vi "fill-lstm-template.vi"() -> ()   [LabVIEW 2020]
uses:
  <vilib>/Analysis/7linalg.llb/Real Transpose Matrix.vi
  <vilib>/Analysis/NI_AALPro.lvlib
panel:
  in  "weight path":path
  in  "name":string
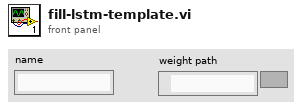
[diagram p1: front panel]
types:
  T1 = typedef "NI_Matrix.lvlib/RealMatrix.ctl" = dbl[][]
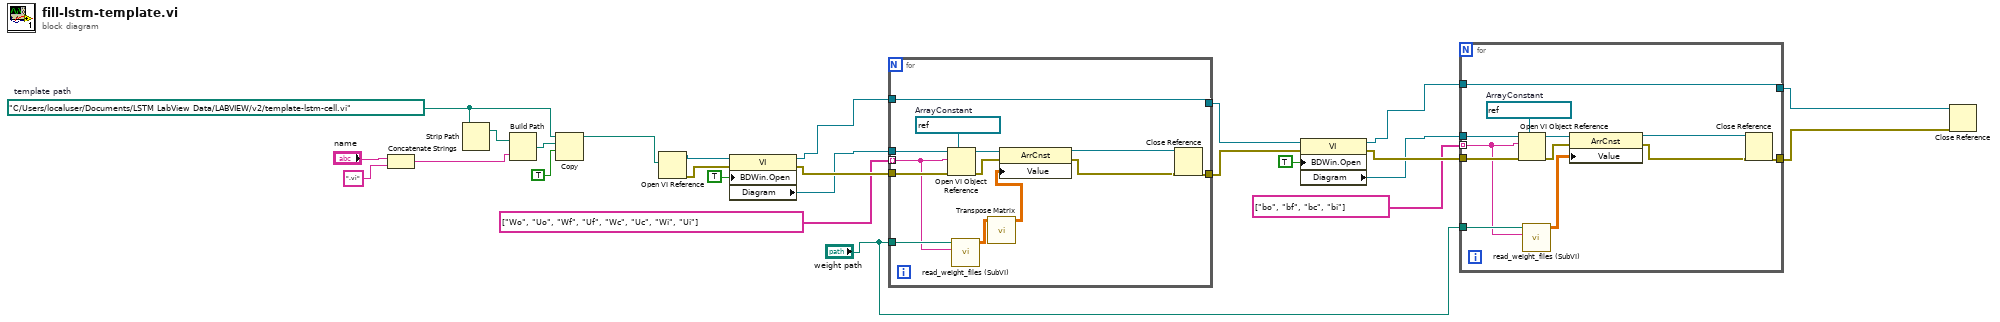
[diagram p0: block diagram]
diagram:
  w18 = path "C:/Users/localuser/Documents/LSTM LabView Data/LABVIEW/v2/template-lstm-cell.vi"  # template path
  n1 = Concatenate Strings("name", ".vi") -> (w20:string)
  n2 = Strip Path(path=w18) -> (stripped path=w23:path)  [unwired: 1 out]
  n3 = Build Path(base path=w23, name or relative path=w20) -> (appended path=w19:path)
  n4 = Copy(9:TRUE, 10:w19, 11:w18) -> (3:w14:path)  [unwired: 2 in, 2 out]
  n5 = Open VI Reference(vi path=w14) -> (vi reference=w16:refnum<vi>, error out=w15:errorcluster)  [unwired: 5 in]
  n6 = property class="VI"(reference=w16, error in=w15, "BDWin.Open"=TRUE) -> (reference out=w12:refnum<vi>, error out=w24:errorcluster, "Diagram"=w13:refnum<vi>)
  n7 = for {
    tunnel: w24 -> [w38]
    tunnel: w13 -> [w37]
    tunnel: string[] ["Wo", "Uo", "Wf", "Uf", "Wc", "Uc", "Wi", "Ui"] -> [w32] mode=indexing
    tunnel: [w30] -> w5
    tunnel: "weight path" -> [w33]
    tunnel: [w31] -> w6
    tunnel: w12 -> [w31]
    w36 = refnum<vi> refnum  # ArrayConstant
    n8 = Open VI Object Reference(7:w36, 8:w38, 10:w32, 11:w37) -> (0:w34:errorcluster, 3:w35:refnum<vi>)
    n9 = call "read_weight_files (SubVI).vi"("weight file name"=w32, "weights path"=w33) -> ("all rows"=w27:dbl[][])  [unwired: 9 in]
    n10 = call-poly <vilib>:"Transpose Matrix.vi"("Input Matrix"=w27) -> ("Matrix Transpose"=w26:T1)  [unwired: 9 in, 1 out]
    n11 = property class="ArrCnst"(reference=w35, error in=w34, "Value"=w26) -> (reference out=w29:refnum<vi>, error out=w28:errorcluster)
    n12 = Close Reference(reference=w29, error in (no error)=w28) -> (error out=w30:errorcluster)
  }
  n13 = property class="VI"(reference=w6, error in=w5, "BDWin.Open"=TRUE) -> (reference out=w7:refnum<vi>, error out=w9:errorcluster, "Diagram"=w8:refnum<vi>)
  n14 = for {
    tunnel: w9 -> [w50]
    tunnel: w8 -> [w49]
    tunnel: string[] ["bo", "bf", "bc", "bi"] -> [w44] mode=indexing
    tunnel: [w42] -> w2
    tunnel: "weight path" -> [w45]
    tunnel: [w43] -> w3
    tunnel: w7 -> [w43]
    w48 = refnum<vi> refnum  # ArrayConstant
    n15 = Open VI Object Reference(7:w48, 8:w50, 10:w44, 11:w49) -> (0:w46:errorcluster, 3:w47:refnum<vi>)
    n16 = call "read_weight_files (SubVI).vi"("weight file name"=w44, "weights path"=w45) -> ("all rows"=w39:dbl[][])  [unwired: 9 in]
    n17 = property class="ArrCnst"(reference=w47, error in=w46, "Value"=w39) -> (reference out=w41:refnum<vi>, error out=w40:errorcluster)
    n18 = Close Reference(reference=w41, error in (no error)=w40) -> (error out=w42:errorcluster)
  }
  n19 = Close Reference(reference=w3, error in (no error)=w2) -> ()  [unwired: 1 out]
